vi "Get Named Sorted Elements.vi"(10 "names":string[](array[string]), 11 "tokens":cluster{"token type":T1, "Type Definition":T2}[](array[cluster])) -> (3 "sorted info":T4(array[cluster]))   [LabVIEW 2019]
uses:
  <vilib>/MultiError/TokenizeJSON/JSON Token Values.ctl
  <vilib>/MultiError/Errors Cluster Multiple Errors/JSON Token Descriptor.ctl
  <vilib>/MultiError/TokenizeJSON/JSON Raw Token Values.ctl
  <vilib>/MultiError/TokenizeJSON/Multi Error Cluster.lvlib
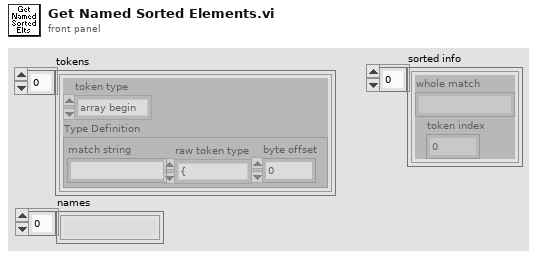
[diagram p1: front panel]
types:
  T1 = typedef "Multi Error Cluster.lvlib/JSON Token Values.ctl" = enum32{"array begin", "array end", "object begin", "object end", "value", "invalid", "name"}
  T2 = typedef "Multi Error Cluster.lvlib/JSON Token Descriptor.ctl" = cluster{"match string":string, "raw token type":T3, "byte offset ":i32}
  T3 = typedef "Multi Error Cluster.lvlib/JSON Raw Token Values.ctl" = enum32{"{", "}", "[", "]", ",", ":", "\"", "number", "string", "true", "false", "null", "invalid"}
  T4 = cluster{"whole match":string, "token index":i32}[]
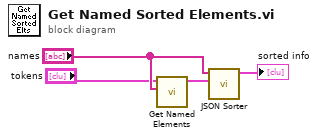
[diagram p0: block diagram]
diagram:
  n1 = call <vilib>:"Get Named Elements.vi"("names"="names", "tokens"="tokens") -> ("Found Token Info"=w2:T4)  [unwired: 9 in]
  n2 = call "JSON Sorter.vi"("Found Token Info"=w2, "names"="names") -> ("Output"=→"sorted info":T4)  [unwired: 9 in]
